vi "p2.vi"() -> ()   [LabVIEW 2025, in "d7.lvlib"]
uses:
  d7.lvlib
  <vilib>/regexp/Match Regular Expression.xnode
  AOC/AOC.lvlib
panel:
  out "Answer":u64=1141028
  in  "Example":string="123 -> x\n456 -> y\nx AND y -> d\nx OR y -> e\nx LSHIFT 2 -> f\ny RSHIFT 2 -> g\nNOT x -> h\nNOT y -> i"
  in  "Example 2":bool=TRUE
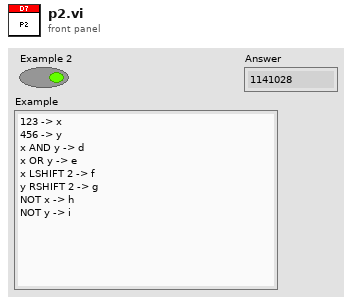
[diagram p1: front panel]
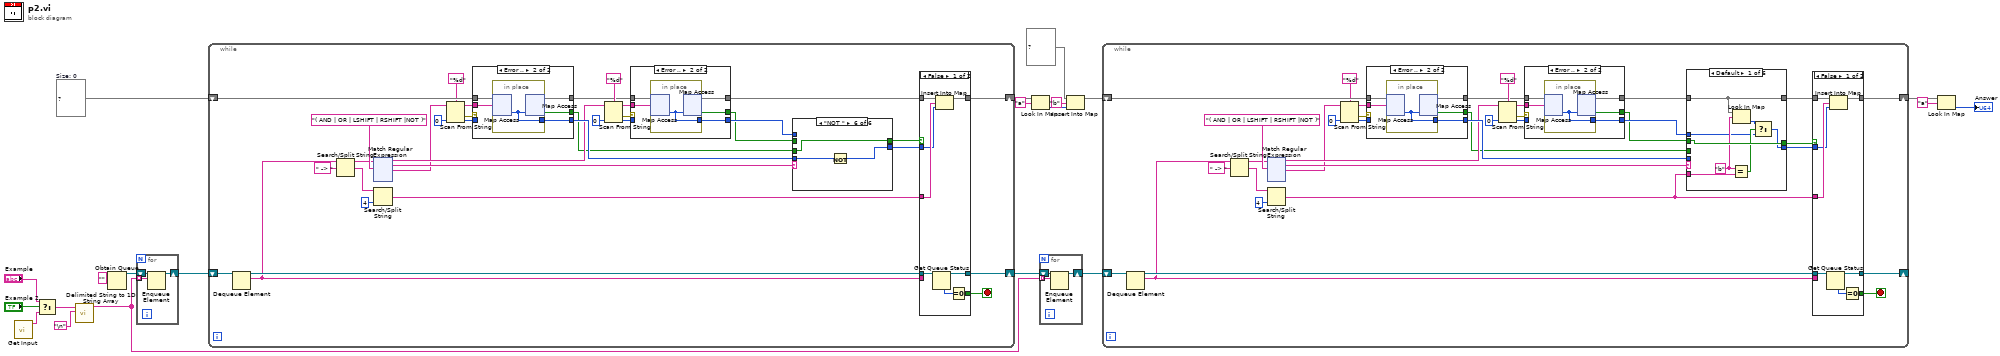
[diagram p0: block diagram]
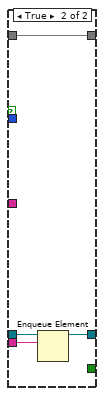
[diagram p2: hidden frame]
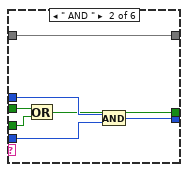
[diagram p3: hidden frame]
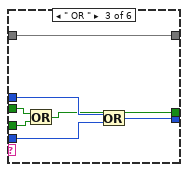
[diagram p4: hidden frame]
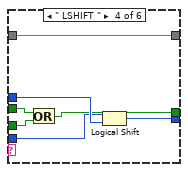
[diagram p5: hidden frame]
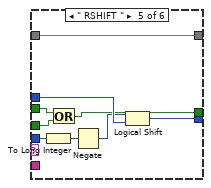
[diagram p6: hidden frame]
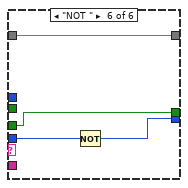
[diagram p7: hidden frame]
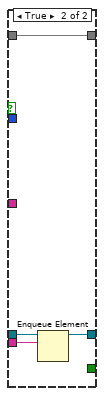
[diagram p10: hidden frame]
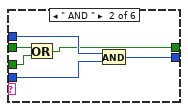
[diagram p12: hidden frame]
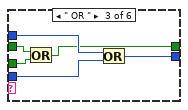
[diagram p13: hidden frame]
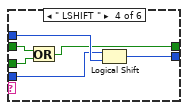
[diagram p14: hidden frame]
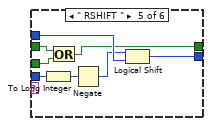
[diagram p15: hidden frame]
diagram:
  w16 = map{string, u16} {}  # Size: 0
  n1 = call "Get Input.vi"() -> ("Input"=w21:string)  [unwired: 11 in]
  n2 = Select(t="Example", s="Example 2", f=w21) -> (s? t:f=w18:string)
  n3 = call <vilib>:"Delimited String to 1D String Array.vi"("delimiter"="\n", "delimited string"=w18) -> ("string array"=w4:string[])  [unwired: 9 in]
  n4 = Obtain Queue(element data type="" ("s? t:f")) -> (queue out=w13:refnum<queue>)  [unwired: 4 in, 2 out]
  n5 = for {
    tunnel: w4 -> [w24] mode=indexing
    shift-right: [w22] -> w12
    shift-left: w13 -> [w23]
    n6 = Enqueue Element(queue=w23, element=w24) -> (queue out=w22:refnum<queue>)  [unwired: 2 in, 2 out]
  }
  n7 = while {
    shift-right: [w53] -> w11
    shift-left: w16 -> [w50]
    shift-right: [w31] -> w6
    shift-left: w12 -> [w33]
    stop <- w30 stop-if-true
    n8 = Dequeue Element(queue=w33) -> (queue out=w32:refnum<queue>, element=w25:string)  [unwired: 2 in, 2 out]
    n9 = Search/Split String(string=w25, search string/char (-)=" -> ") -> (substring before match=w57:string, match + rest of string=w55:string)  [unwired: 1 in, 1 out]
    n10 = xnode "Match Regular Expression"("input string"=w57, "regular expression"="( AND | OR | LSHIFT | RSHIFT |NOT )") -> ("before match"=w35:string, "whole match"=w51:string, "after match"=w34:string)  [unwired: 4 in, 2 out]
    n11 = Search/Split String(string=w55, offset (0)=4) -> (match + rest of string=w52:string)  [unwired: 1 in, 2 out]
    n12 = Scan From String(format string="%d", input string=w34, default 1=u16 0 ("default value 14")) -> (remaining string=w44:string, error out=w46:errorcluster, output 1=w45:u16)  [unwired: 2 in, 1 out]
    n13 = case shown="Error .." w46 {
      tunnel: w50 -> [w111 w116]
      tunnel: [w110 w115] -> w49
      tunnel: [w111 w114] -> w38
      tunnel: w44 -> [_ w113]
      tunnel: w45 -> [w110 _]
      tunnel: [_ w112] -> w28
      frame #0 {
      }
      frame #1 {
        n14 = in-place {
          in-place-border: [w117] -> w115
          n15 = in-place-map #1(w116, w113) -> (w117:u16)  [unwired: 1 in, 1 out]
          n16 = in-place-map #1(w117) -> (w114:map{string, u16}, w112:bool)  [unwired: 1 in, 1 out]
        }
      }
    }
    n17 = Scan From String(format string="%d", input string=w35, default 1=u16 0 ("default value 14")) -> (remaining string=w39:string, error out=w41:errorcluster, output 1=w40:u16)  [unwired: 2 in, 1 out]
    n18 = case shown="Error .." w41 {
      tunnel: w38 -> [w103 w108]
      tunnel: [w102 w107] -> w36
      tunnel: [w103 w106] -> w37
      tunnel: w39 -> [_ w105]
      tunnel: w40 -> [w102 _]
      tunnel: [_ w104] -> w27
      frame #0 {
      }
      frame #1 {
        n19 = in-place {
          in-place-border: [w109] -> w107
          n20 = in-place-map #2(w108, w105) -> (w109:u16)  [unwired: 1 in, 1 out]
          n21 = in-place-map #2(w109) -> (w106:map{string, u16}, w104:bool)  [unwired: 1 in, 1 out]
        }
      }
    }
    n22 = case shown="\"NOT \"" w51 {
      tunnel: [w72 w76 w82 w90 w98 w100] -> w29
      tunnel: w49 -> [_ w77 w83 w88 w96 w101]
      tunnel: w36 -> [w72 w78 w84 w89 w97 _]
      tunnel: w28 -> [_ w74 w80 w87 w92 w99]
      tunnel: w27 -> [w71 w75 w81 w86 w93 _]
      tunnel: [w71 w73 w79 w85 w91 w99] -> w26
      frame Default {
      }
      frame " AND " {
        n23 = Or(x=w75, y=w74) -> (x .or. y?=w73:bool)
        n24 = And(x=w78, y=w77) -> (x .and. y?=w76:u16)
      }
      frame " OR " {
        n25 = Or(x=w81, y=w80) -> (x .or. y?=w79:bool)
        n26 = Or(x=w84, y=w83) -> (x .or. y?=w82:u16)
      }
      frame " LSHIFT " {
        n27 = Or(x=w86, y=w87) -> (x .or. y?=w85:bool)
        n28 = Logical Shift(y=w88, x=w89) -> (x << y=w90:u16)
      }
      frame " RSHIFT " {
        n29 = To Long Integer(number=w96) -> (32bit integer=w95:i32)
        n30 = Or(x=w93, y=w92) -> (x .or. y?=w91:bool)
        n31 = Negate(x=w95) -> (-x=w94:i32)
        n32 = Logical Shift(y=w94, x=w97) -> (x << y=w98:u16)
      }
      frame "NOT " {
        n33 = Not(x=w101) -> (.not. x?=w100:u16)
      }
    }
    n34 = case shown="False" w26 {
      tunnel: [w66 w70] -> w53
      tunnel: w52 -> [w65 _]
      tunnel: w37 -> [w64 w70]
      tunnel: w32 -> [w63 w69]
      tunnel: [w62 w68] -> w31
      tunnel: [w61 _] -> w30
      tunnel: w29 -> [w60 _]
      tunnel: w25 -> [_ w67]
      frame False {
        n35 = Get Queue Status(queue=w63) -> (queue out=w62:refnum<queue>, # elements in queue=w59:i32)  [unwired: 2 in, 6 out]
        n36 = Insert Into Map(map in=w64, key=w65, value=w60) -> (map out=w66:map{string, u16})  [unwired: 2 out]
        n37 = Equal To 0?(x=w59) -> (x = 0?=w61:bool)
      }
      frame True {
        n38 = Enqueue Element(queue=w69, element=w67) -> (queue out=w68:refnum<queue>)  [unwired: 2 in, 2 out]
      }
    }
  }
  n39 = Look In Map(map=w11, key="a") -> (value=w9:u16)  [unwired: 1 in, 1 out]
  n40 = for {
    tunnel: w4 -> [w237] mode=indexing
    shift-right: [w235] -> w5
    shift-left: w6 -> [w236]
    n41 = Enqueue Element(queue=w236, element=w237) -> (queue out=w235:refnum<queue>)  [unwired: 2 in, 2 out]
  }
  n42 = Insert Into Map(map in=map{string, u16} {}, key="b", value=w9) -> (map out=w8:map{string, u16})  [unwired: 2 out]
  n43 = while {
    shift-right: [w267] -> w2
    shift-left: w8 -> [w265]
    shift-right: [w247] -> _
    shift-left: w5 -> [w249]
    stop <- w246 stop-if-true
    n44 = Dequeue Element(queue=w249) -> (queue out=w248:refnum<queue>, element=w241:string)  [unwired: 2 in, 2 out]
    n45 = Search/Split String(string=w241, search string/char (-)=" -> ") -> (substring before match=w271:string, match + rest of string=w269:string)  [unwired: 1 in, 1 out]
    n46 = xnode "Match Regular Expression"("input string"=w271, "regular expression"="( AND | OR | LSHIFT | RSHIFT |NOT )") -> ("before match"=w251:string, "whole match"=w266:string, "after match"=w250:string)  [unwired: 4 in, 2 out]
    n47 = Search/Split String(string=w269, offset (0)=4) -> (match + rest of string=w240:string)  [unwired: 1 in, 2 out]
    n48 = Scan From String(format string="%d", input string=w250, default 1=u16 0 ("default value 14")) -> (remaining string=w259:string, error out=w261:errorcluster, output 1=w260:u16)  [unwired: 2 in, 1 out]
    n49 = case shown="Error .." w261 {
      tunnel: w265 -> [w336 w341]
      tunnel: [w335 w340] -> w264
      tunnel: [w336 w339] -> w253
      tunnel: w259 -> [_ w338]
      tunnel: w260 -> [w335 _]
      tunnel: [_ w337] -> w244
      frame #0 {
      }
      frame #1 {
        n50 = in-place {
          in-place-border: [w342] -> w340
          n51 = in-place-map #3(w341, w338) -> (w342:u16)  [unwired: 1 in, 1 out]
          n52 = in-place-map #3(w342) -> (w339:map{string, u16}, w337:bool)  [unwired: 1 in, 1 out]
        }
      }
    }
    n53 = Scan From String(format string="%d", input string=w251, default 1=u16 0 ("default value 14")) -> (remaining string=w254:string, error out=w256:errorcluster, output 1=w255:u16)  [unwired: 2 in, 1 out]
    n54 = case shown="Error .." w256 {
      tunnel: w253 -> [w328 w333]
      tunnel: [w327 w332] -> w252
      tunnel: [w328 w331] -> w239
      tunnel: w254 -> [_ w330]
      tunnel: w255 -> [w327 _]
      tunnel: [_ w329] -> w243
      frame #0 {
      }
      frame #1 {
        n55 = in-place {
          in-place-border: [w334] -> w332
          n56 = in-place-map #4(w333, w330) -> (w334:u16)  [unwired: 1 in, 1 out]
          n57 = in-place-map #4(w334) -> (w331:map{string, u16}, w329:bool)  [unwired: 1 in, 1 out]
        }
      }
    }
    n58 = case shown="Default" w266 {
      tunnel: [w285 w297 w304 w313 w322 w325] -> w245
      tunnel: w264 -> [_ w298 w305 w311 w320 w326]
      tunnel: w252 -> [w286 w299 w306 w312 w321 _]
      tunnel: w244 -> [_ w295 w302 w310 w316 w324]
      tunnel: w243 -> [w292 w296 w303 w309 w317 _]
      tunnel: [w292 w294 w301 w308 w315 w324] -> w242
      tunnel: w240 -> [w291 _ _ _ _ _]
      tunnel: w239 -> [w288 w293 w300 w307 w314 w323]
      tunnel: [w288 w293 w300 w307 w314 w323] -> w238
      frame Default {
        w290 = "b" ("x")
        n59 = Equal?(x=w290, y=w291) -> (x = y?=w289:bool)
        n60 = Look In Map(map=w288, key=w290) -> (value=w287:u16)  [unwired: 1 in, 1 out]
        n61 = Select(t=w287, s=w289, f=w286) -> (s? t:f=w285:u16)
      }
      frame " AND " {
        n62 = Or(x=w296, y=w295) -> (x .or. y?=w294:bool)
        n63 = And(x=w299, y=w298) -> (x .and. y?=w297:u16)
      }
      frame " OR " {
        n64 = Or(x=w303, y=w302) -> (x .or. y?=w301:bool)
        n65 = Or(x=w306, y=w305) -> (x .or. y?=w304:u16)
      }
      frame " LSHIFT " {
        n66 = Or(x=w309, y=w310) -> (x .or. y?=w308:bool)
        n67 = Logical Shift(y=w311, x=w312) -> (x << y=w313:u16)
      }
      frame " RSHIFT " {
        n68 = To Long Integer(number=w320) -> (32bit integer=w319:i32)
        n69 = Or(x=w317, y=w316) -> (x .or. y?=w315:bool)
        n70 = Negate(x=w319) -> (-x=w318:i32)
        n71 = Logical Shift(y=w318, x=w321) -> (x << y=w322:u16)
      }
      frame "NOT " {
        n72 = Not(x=w326) -> (.not. x?=w325:u16)
      }
    }
    n73 = case shown="False" w242 {
      tunnel: [w280 w284] -> w267
      tunnel: w240 -> [w279 _]
      tunnel: w238 -> [w278 w284]
      tunnel: w248 -> [w277 w283]
      tunnel: [w276 w282] -> w247
      tunnel: [w275 _] -> w246
      tunnel: w245 -> [w274 _]
      tunnel: w241 -> [_ w281]
      frame False {
        n74 = Get Queue Status(queue=w277) -> (queue out=w276:refnum<queue>, # elements in queue=w273:i32)  [unwired: 2 in, 6 out]
        n75 = Insert Into Map(map in=w278, key=w279, value=w274) -> (map out=w280:map{string, u16})  [unwired: 2 out]
        n76 = Equal To 0?(x=w273) -> (x = 0?=w275:bool)
      }
      frame True {
        n77 = Enqueue Element(queue=w283, element=w281) -> (queue out=w282:refnum<queue>)  [unwired: 2 in, 2 out]
      }
    }
  }
  n78 = Look In Map(map=w2, key="a") -> (value=→"Answer":u16)  [unwired: 1 in, 1 out]
